vi "Read Msg Input.vi"(10 "Msg Input":refnum<class "Msg Input.lvclass">) -> (1 "Error":errorcluster, 2 "Actor":refnum<class "Actor.lvclass">, 4 "Teller":refnum<class "Teller.lvclass">)   [LabVIEW 2020, in "jettl.lvlib" / "Stopped jettl Msg.lvlib" / "Stopped Msg Input.lvlib"]
uses:
  Stopped Msg Input.lvlib
  Actor/Actor.lvclass
  Teller/Teller.lvclass
  Msg Input/Msg Input.lvclass
  Stopped Msg Input/Stopped Msg Input.lvclass
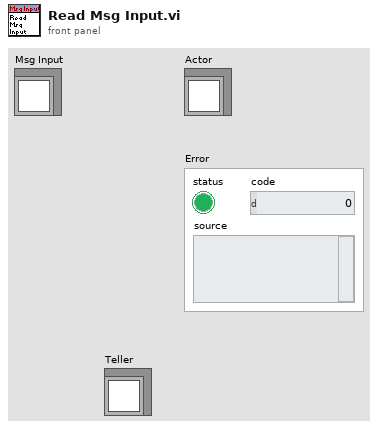
[diagram p1: front panel]
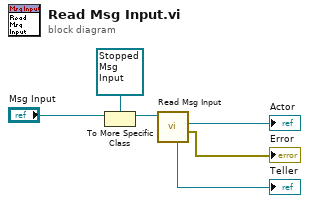
[diagram p0: block diagram]
diagram:
  n1 = To More Specific Class(target class=refnum<class "Stopped Msg Input.lvclass"> refnum ("jettl.lvlib:Stopped jettl Msg.lvlib:Stopped Msg Input.lvlib:Stopped Msg Input.lvclass"), reference="Msg Input") -> (specific class reference=w5:refnum<class "Stopped Msg Input.lvclass">)  [unwired: 1 in, 1 out]
  n2 = call "Read Msg Input.vi"("Stopped Msg Input in"=w5) -> ("Error"=→"Error":errorcluster, "Actor"=→"Actor":refnum<class "Actor.lvclass">, "Teller"=→"Teller":refnum<class "Teller.lvclass">)  [unwired: 8 in]
